vi "Example - Configure Host DMA Buffer Size.vi"(0 "fpga reference":refnum<k20>, 1 "host DMA buffer size (samples)":u32, 2 "host DMA buffer num of blocks":u32=1, 3 "host DMA buffer block size divisor (bytes)":u32=1, 5 "error in (no error)":errorcluster) -> (15 "actual host DMA buffer size (samples)":u32, 16 "actual host DMA buffer size (elements)":u32, 17 "transfer quantum size (samples)":u64, 18 "transfer quantum size (elements)":u64, 19 "error out":errorcluster)   [LabVIEW 2021, in "Disk Streaming.lvclass"]
uses:
  Disk Streaming.lvclass
  <vilib>/Utility/error.llb/Error Cluster From Error Code.vi
  <vilib>/rvi/interface/common/niFpgaWaitOnOcc.vi
  <vilib>/rvi/interface/nirviMethod/nirviMethod.xnode
  <vilib>/ErrorRing/Error Ring.xnode
  <vilib>/rvi/errors/niLvFpgaMergeErrorWithErrorCode.vi
  <vilib>/FPGAPlugInAG/Dynamic/niLvFpga_StartFifo_Dynamic.vi
  <vilib>/FPGAPlugInAG/Dynamic/niLvFpga_ConfigureFifo_Dynamic.vi
  <vilib>/gmath/NI_Gmath.lvlib
  <vilib>/FPGAPlugInAG/Dynamic/niLvFpga_StopFifo_Dynamic.vi
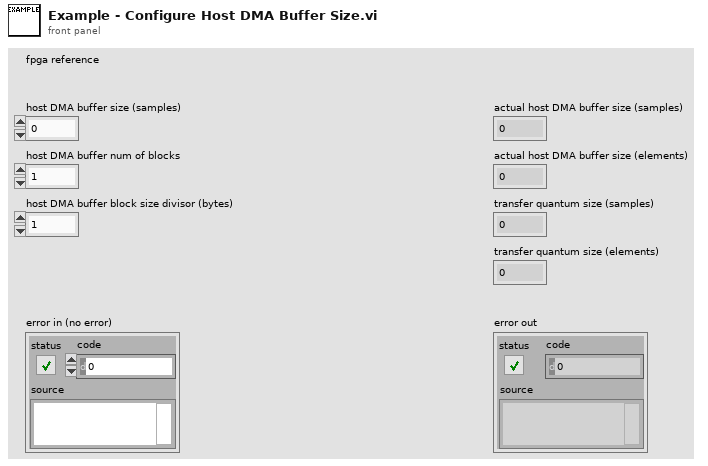
[diagram p1: front panel]
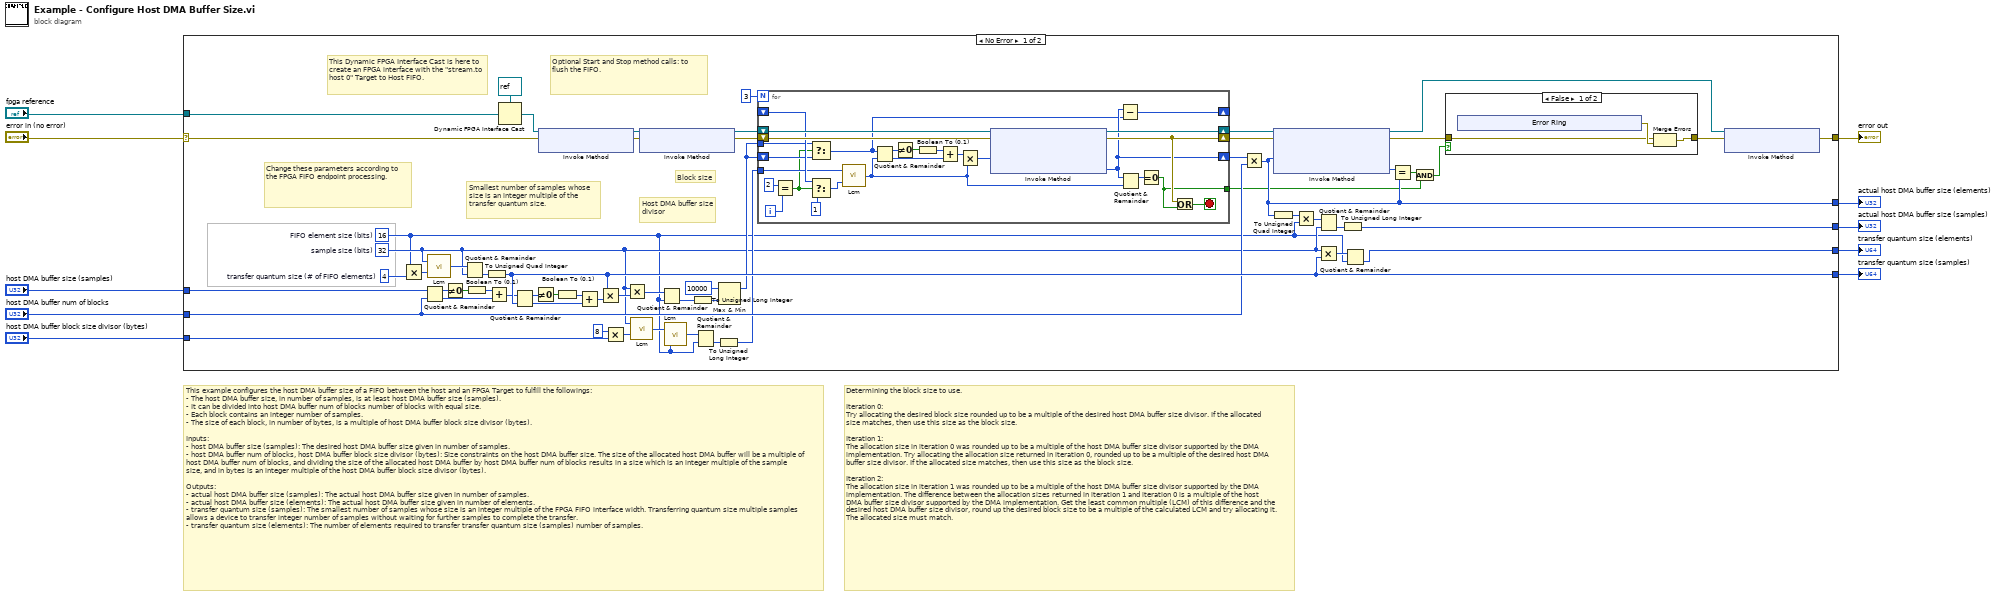
[diagram p0: block diagram]
diagram:
  # "Determining the block size to use.\n\nIteration 0:\nTry allocating the desired block size rounded up to be a multiple of the desired host DMA buffer size divisor. If the allocated size matches, then use this size as the block size.\n\nIteration 1:\nThe allocation size in iteration 0 was rounded up to be a multiple of the host DMA buffer size divisor supported by the DMA implementation. Try allocating the allocation size returned in iteration 0, rounded up to be a multiple of the desired host DMA buffer size divisor. If the allocated size matches, then use this size as the block size.\n\nIteration 2:\nThe allocation size in iteration 1 was rounded up to be a multiple of the host DMA buffer size divisor supported by the DMA implementation. The difference between the allocation sizes returned in iteration 1 and iteration 0 is a multiple of the host DMA buffer size divisor supported by the DMA implementation. Get the least common multiple (LCM) of this difference and the desired host DMA buffer size divisor, round up the desired block size to be a multiple of the calculated LCM and try allocating it. The allocated size must match."
  # "This example configures the host DMA buffer size of a FIFO between the host and an FPGA Target to fulfill the followings:\n- The host DMA buffer size, in number of samples, is at least host DMA buffer size (samples).\n- It can be divided into host DMA buffer num of blocks number of blocks with equal size.\n- Each block contains an integer number of samples.\n- The size of each block, in number of bytes, is a multiple of host DMA buffer block size divisor (bytes).\n\nInputs:\n- host DMA buffer size (samples): The desired host DMA buffer size given in number of samples.\n- host DMA buffer num of blocks, host DMA buffer block size divisor (bytes): Size constraints on the host DMA buffer size. The size of the allocated host DMA buffer will be a multiple of host DMA buffer num of blocks, and dividing the size of the allocated host DMA buffer by host DMA buffer num of blocks results in a size which is an integer multiple of the sample size, and in bytes is an integer multiple of the host DMA buffer block size divisor (bytes).\n\nOutputs:\n- actual host DMA buffer size (samples): The actual host DMA buffer size given in number of samples.\n- actual host DMA buffer size (elements): The actual host DMA buffer size given in number of elements.\n- transfer quantum size (samples): The smallest number of samples whose size is an integer multiple of the FPGA FIFO interface width. Transferring quantum size multiple samples allows a device to transfer integer number of samples without waiting for further samples to complete the transfer.\n- transfer quantum size (elements): The number of elements required to transfer transfer quantum size (samples) number of samples."
  n1 = case shown="No Error" "error in (no error)" {
    selector: "error in (no error)" -> [w13 w105]
    tunnel: [w11 w105] -> w9
    tunnel: "host DMA buffer size (samples)" -> [w69 _]
    tunnel: [w68 _] -> w7
    tunnel: [w67 _] -> w6
    tunnel: [w66 _] -> w5
    tunnel: [w65 _] -> w4
    tunnel: "host DMA buffer num of blocks" -> [w64 _]
    tunnel: "host DMA buffer block size divisor (bytes)" -> [w63 _]
    tunnel: "fpga reference" -> [w12 _]
    frame No Error {
      w15 = 4  # transfer quantum size (# of FIFO elements)
      w16 = 16  # FIFO element size (bits)
      w17 = 32  # sample size (bits)
      # "Host DMA buffer size divisor"
      # "Block size"
      # "Optional Start and Stop method calls: to flush the FIFO."
      # "Change these parameters according to the FPGA FIFO endpoint processing."
      # "This Dynamic FPGA Interface Cast is here to create an FPGA interface with the \"stream.to host 0\" Target to Host FIFO."
      # "Smallest number of samples whose size is an integer multiple of the transfer quantum size."
      n2 = Multiply(x=w16, y=w15) -> (x*y=w34:i32)
      n3 = Quotient & Remainder(x=w69, y=w64) -> (x-y*floor(x/y)=w38:u32, floor(x/y)=w35:u32)
      n4 = call <vilib>:"Lcm.vi"("y"=w34, "x"=w17) -> ("lcm(x,y)"=w18:i64)
      n5 = Not Equal To 0?(x=w38) -> (x != 0?=w37:bool)
      n6 = Quotient & Remainder(x=w18, y=w17) -> (floor(x/y)=w21:i64)  [unwired: 1 out]
      n7 = Boolean To (0,1)(Boolean=w37) -> (0, 1=w36:i16)
      n8 = To Unsigned Quad Integer(1:w21) -> (0:w66:u64)
      n9 = Add(x=w36, y=w35) -> (x+y=w28:u32)
      n10 = Dynamic FPGA Interface Cast(Session In=refnum<k20> refnum ("FPGA Interface"), Type=w12) -> (Session Out=w14:refnum<k20>)
      n11 = Quotient & Remainder(x=w28, y=w66) -> (x-y*floor(x/y)=w29:u64, floor(x/y)=w32:u64)
      n12 = Not Equal To 0?(x=w29) -> (x != 0?=w30:bool)
      n13 = xnode "Invoke Method"("FPGA VI Reference In"=w14, "error in"=w13) -> ("FPGA VI Reference Out"=w24:refnum<k20>, "error out"=w25:errorcluster)
      n14 = Boolean To (0,1)(Boolean=w30) -> (0, 1=w31:i16)
      n15 = Add(x=w31, y=w32) -> (x+y=w33:u64)
      n16 = Multiply(x=w66, y=w33) -> (x*y=w20:u64)
      n17 = Multiply(x=u32 8 ("y"), y=w63) -> (x*y=w59:u32)
      n18 = Multiply(x=w17, y=w20) -> (x*y=w56:u64)
      n19 = call <vilib>:"Lcm.vi"("y"=w59, "x"=w17) -> ("lcm(x,y)"=w58:i64)
      n20 = xnode "Invoke Method"("FPGA VI Reference In"=w24, "error in"=w25) -> ("FPGA VI Reference Out"=w22:refnum<k20>, "error out"=w23:errorcluster)
      n21 = Quotient & Remainder(x=w56, y=w16) -> (floor(x/y)=w27:u64)  [unwired: 1 out]
      n22 = call <vilib>:"Lcm.vi"("y"=w16, "x"=w58) -> ("lcm(x,y)"=w57:i64)
      n23 = To Unsigned Long Integer(number=w27) -> (unsigned 32bit integer=w26:u32)
      n24 = Quotient & Remainder(x=w57, y=w16) -> (floor(x/y)=w50:i64)  [unwired: 1 out]
      n25 = To Unsigned Long Integer(number=w50) -> (unsigned 32bit integer=w54:u32)
      n26 = Max & Min(x=u32 10000, y=w26) -> (max(x,y)=w39:u32)  [unwired: 1 out]
      n27 = for {
        N: 3 -> [_]
        shift-right: [w102] -> w48
        shift-left: w22 -> [w101]
        shift-right: [w103] -> w47
        shift-left: w23 -> [w104]
        tunnel: w54 -> [w87]
        tunnel: [w100] -> w44
        shift-right: [w93] -> w49
        shift-left: w39 -> [w84]
        shift-right: [w92] -> _
        shift-left: _ -> [w90]
        tunnel: w39 -> [w81]
        i -> [w86]
        stop <- w80 stop-if-true
        n28 = Equal?(x=2, y=w86) -> (x = y?=w83:bool)
        n29 = Select(t=w81, s=w83, f=w84) -> (s? t:f=w82:u32)
        n30 = Select(t=w90, s=w83, f=u32 1) -> (s? t:f=w88:u32)
        n31 = call <vilib>:"Lcm.vi"("y"=w88, "x"=w87) -> ("lcm(x,y)"=w79:i64)
        n32 = Quotient & Remainder(x=w82, y=w79) -> (x-y*floor(x/y)=w99:i64, floor(x/y)=w96:i64)
        n33 = Not Equal To 0?(x=w99) -> (x != 0?=w98:bool)
        n34 = Boolean To (0,1)(Boolean=w98) -> (0, 1=w97:i16)
        n35 = Add(x=w97, y=w96) -> (x+y=w95:i64)
        n36 = Multiply(x=w95, y=w79) -> (x*y=w94:i64)
        n37 = xnode "Invoke Method"("FPGA VI Reference In"=w101, "error in"=w104, "Requested Depth"=w94) -> ("FPGA VI Reference Out"=w102:refnum<k20>, "error out"=w103:errorcluster, "Actual Depth"=w93:u32)
        n38 = Subtract(x=w93, y=w82) -> (x-y=w92:u32)
        n39 = Quotient & Remainder(x=w93, y=w79) -> (x-y*floor(x/y)=w85:i64)  [unwired: 1 out]
        n40 = Equal To 0?(x=w85) -> (x = 0?=w100:bool)
        n41 = Or(x=w103, y=w100) -> (x .or. y?=w80:bool)
      }
      n42 = Multiply(x=w49, y=w64) -> (x*y=w68:u32)
      n43 = To Unsigned Quad Integer(1:w68) -> (0:w53:u64)
      n44 = xnode "Invoke Method"("FPGA VI Reference In"=w48, "error in"=w47, "Requested Depth"=w68) -> ("FPGA VI Reference Out"=w40:refnum<k20>, "error out"=w43:errorcluster, "Actual Depth"=w46:u32)
      n45 = Multiply(x=w53, y=w16) -> (x*y=w52:u64)
      n46 = Multiply(x=w17, y=w66) -> (x*y=w19:u64)
      n47 = Quotient & Remainder(x=w52, y=w17) -> (floor(x/y)=w51:u64)  [unwired: 1 out]
      n48 = To Unsigned Long Integer(number=w51) -> (unsigned 32bit integer=w67:u32)
      n49 = Quotient & Remainder(x=w19, y=w16) -> (floor(x/y)=w65:u64)  [unwired: 1 out]
      n50 = Equal?(x=w46, y=w68) -> (x = y?=w45:bool)
      n51 = And(x=w45, y=w44) -> (x .and. y?=w42:bool)
      n52 = case shown="False" w42 {
        tunnel: w43 -> [w71 w78]
        tunnel: [w70 w78] -> w41
        frame False {
          n53 = xnode "Error Ring"() -> ("error out"=w72:errorcluster)
          n54 = Merge Errors(w71, w72) -> (w70:errorcluster)
        }
        frame True {
        }
      }
      n55 = xnode "Invoke Method"("FPGA VI Reference In"=w40, "error in"=w41) -> ("error out"=w11:errorcluster)  [unwired: 1 out]
    }
    frame Error {
    }
  }
  "error out" <- w9
  "actual host DMA buffer size (elements)" <- w7
  "actual host DMA buffer size (samples)" <- w6
  "transfer quantum size (samples)" <- w5
  "transfer quantum size (elements)" <- w4
